vi "Init After.vi"(11 "UI References":refnum<vi>[](array[refnum])) -> ()   [LabVIEW 2019, in "LSS.lvlib"]
doc: "Intiailize the front panel of the example using LSS.\n\n<b>Inputs:</b>\n<b>UI References</b> - Array of objects from the front panel of the example."
uses:
  LSS.lvlib
  <vilib>/Utility/miscctls.llb/LVBoundsTypeDef.ctl
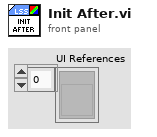
[diagram p1: front panel]
types:
  T1 = typedef "LVBoundsTypeDef.ctl" = cluster{"Width":u32, "Height":u32}
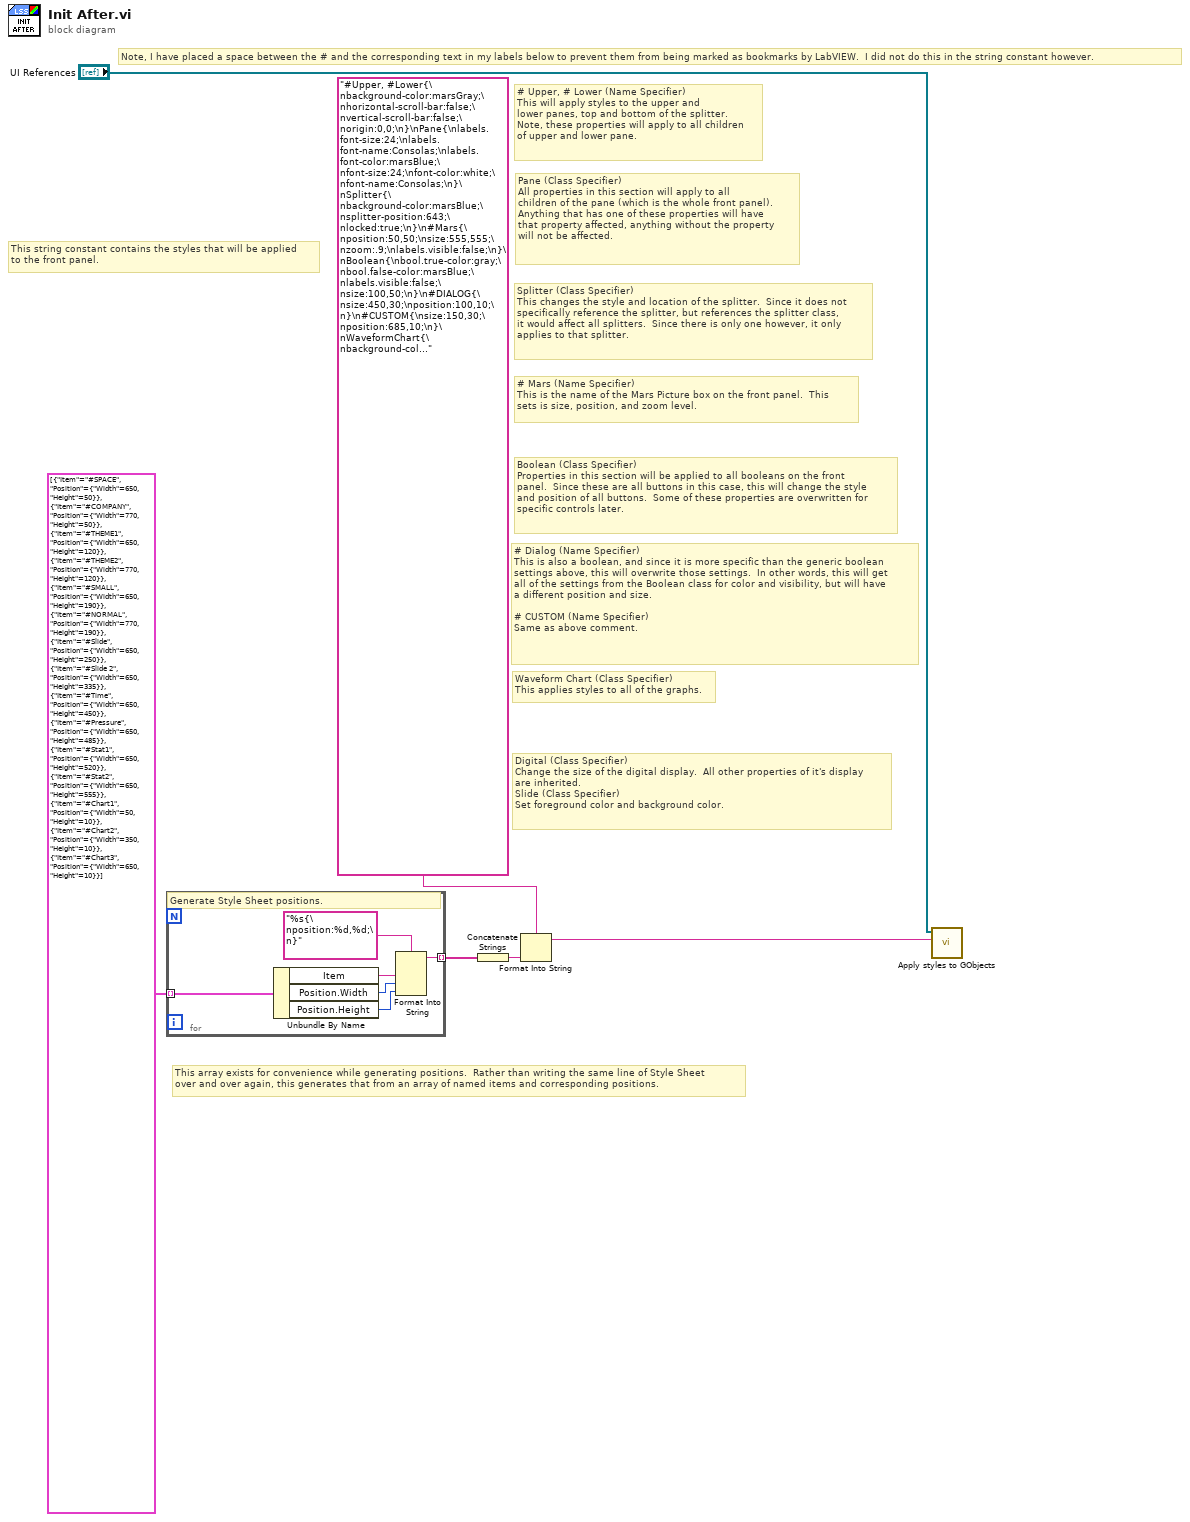
[diagram p0: block diagram]
diagram:
  # "Digital (Class Specifier)\nChange the size of the digital display.  All other properties of it's display\nare inherited.\nSlide (Class Specifier)\nSet foreground color and background color."
  # "Waveform Chart (Class Specifier)\nThis applies styles to all of the graphs."
  # "# Dialog (Name Specifier)\nThis is also a boolean, and since it is more specific than the generic boolean\nsettings above, this will overwrite those settings.  In other words, this will get\nall of the settings from the Boolean class for color and visibility, but will have\na different position and size.\n\n# CUSTOM (Name Specifier)\nSame as above comment."
  # "Boolean (Class Specifier)\nProperties in this section will be applied to all booleans on the front\npanel.  Since these are all buttons in this case, this will change the style\nand position of all buttons.  Some of these properties are overwritten for\nspecific controls later."
  # "# Mars (Name Specifier)\nThis is the name of the Mars Picture box on the front panel.  This\nsets is size, position, and zoom level."
  # "Splitter (Class Specifier)\nThis changes the style and location of the splitter.  Since it does not\nspecifically reference the splitter, but references the splitter class,\nit would affect all splitters.  Since there is only one however, it only \napplies to that splitter."
  # "Pane (Class Specifier)\nAll properties in this section will apply to all\nchildren of the pane (which is the whole front panel).\nAnything that has one of these properties will have\nthat property affected, anything without the property\nwill not be affected."
  # "Note, I have placed a space between the # and the corresponding text in my labels below to prevent them from being marked as bookmarks by LabVIEW.  I did not do this in the string constant however."
  # "# Upper, # Lower (Name Specifier)\nThis will apply styles to the upper and\nlower panes, top and bottom of the splitter.\nNote, these properties will apply to all children\nof upper and lower pane."
  # "This string constant contains the styles that will be applied\nto the front panel."
  # "This array exists for convenience while generating positions.  Rather than writing the same line of Style Sheet\nover and over again, this generates that from an array of named items and corresponding positions."
  n1 = for {
    tunnel: cluster{"Item":string, "Position":T1}[] [{"Item"="#SPACE", "Position"={"Width"=650, "Height"=50}}, {"Item"="#COMPANY", "Position"={"Width"=770, "Height"=50}}, {"Item"="#THEME1", "Position"={"Width"=650, "Height"=120}}, {"Item"="#THEME2", "Position"={"Width"=770, "Height"=120}}, {"Item"="#SMALL", "Position"={"Width"=650, "Height"=190}}, {"Item"="#NORMAL", "Position"={"Width"=770, "Height"=190}}, {"Item"="#Slide", "Position"={"Width"=650, "Height"=250}}, {"Item"="#Slide 2", "Position"={"Width"=650, "Height"=335}}, {"Item"="#Time", "Position"={"Width"=650, "Height"=450}}, {"Item"="#Pressure", "Position"={"Width"=650, "Height"=485}}, {"Item"="#Stat1", "Position"={"Width"=650, "Height"=520}}, {"Item"="#Stat2", "Position"={"Width"=650, "Height"=555}}, {"Item"="#Chart1", "Position"={"Width"=50, "Height"=10}}, {"Item"="#Chart2", "Position"={"Width"=350, "Height"=10}}, {"Item"="#Chart3", "Position"={"Width"=650, "Height"=10}}] -> [w12] mode=indexing
    tunnel: [w7] -> w3 mode=indexing
    # "Generate Style Sheet positions."
    n2 = Unbundle By Name(w12) -> ("Item"=w10:string, "Position.Width"=w9:u32, "Position.Height"=w8:u32)
    n3 = Format Into String(format string="%s{\nposition:%d,%d;\n}", w10, w9, w8) -> (resulting string=w7:string)  [unwired: 2 in, 1 out]
  }
  n4 = Concatenate Strings(w3) -> (w2:string)
  n5 = Format Into String(format string="#Upper, #Lower{\nbackground-color:marsGray;\nhorizontal-scroll-bar:false;\nvertical-scroll-bar:false;\norigin:0,0;\n}\nPane{\nlabels.font-size:24;\nlabels.font-name:Consolas;\nlabels.font-color:marsBlue;\nfont-size:24;\nfont-color:white;\nfont-name:Consolas;\n}\nSplitter{\nbackground-color:marsBlue;\nsplitter-position:643;\nlocked:true;\n}\n#Mars{\nposition:50,50;\nsize:555,555;\nzoom:.9;\nlabels.visible:false;\n}\nBoolean{\nbool.true-color:gray;\nbool.false-color:marsBlue;\nlabels.visible:false;\nsize:100,50;\n}\n#DIALOG{\nsize:450,30;\nposition:100,10;\n}\n#CUSTOM{\nsize:150,30;\nposition:685,10;\n}\nWaveformChart{\nbackground-color:gray;\ngraph.frame-color:transparent;\nplot-color:0,marsBlue;\nlabels.font-color:white;\n}\nDigital{\nsize:100;\n}\nSlide{\nbackground-color:gray;\ncolor:marsBlue;\n}\n%s" ("String"), w2) -> (resulting string=w1:string)  [unwired: 2 in, 1 out]
  n6 = call "Apply styles to GObjects.vi"("Style Sheet"=w1, "Front Panel Objects"="UI References") -> ()  [unwired: 8 in, 2 out]
